vi "get FPS.vi"(8 "error in (no error)":errorcluster, 11 "Thorcam in":refnum<class "Thorcam.lvclass">) -> (0 "error out":errorcluster, 3 "Thorcam out":refnum<class "Thorcam.lvclass">)   [LabVIEW 2012, in "Thorcam.lvclass"]
uses:
  Thorcam.lvclass
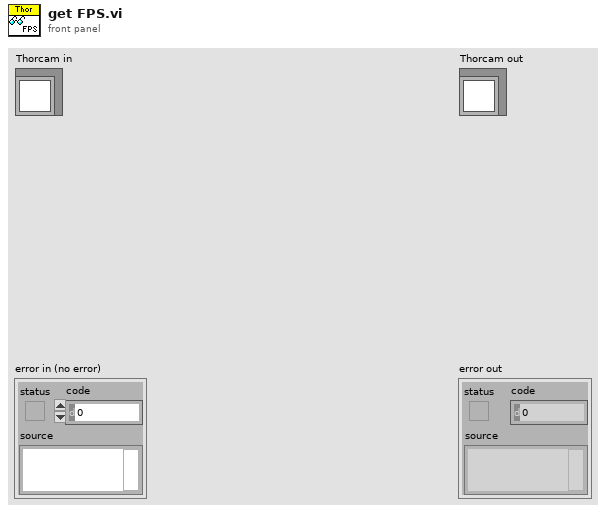
[diagram p1: front panel]
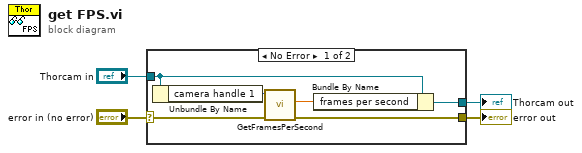
[diagram p0: block diagram]
diagram:
  n1 = case shown="No Error" "error in (no error)" {
    selector: "error in (no error)" -> [w9 w12]
    tunnel: [w8 w12] -> w3
    tunnel: [w6 w11] -> w1
    tunnel: "Thorcam in" -> [w7 w11]
    frame No Error {
      n2 = Unbundle By Name(w7) -> ("camera handle 1"=w10:u32)
      n3 = call <instrlib>:"GetFramesPerSecond.vi"("error in"=w9, "Camera Handle In"=w10) -> ("error out"=w8:errorcluster, "FPS"=w5:dbl)  [unwired: 7 in, 1 out]
      n4 = Bundle By Name(cluster=w7, "frames per second"=w5) -> (w6:refnum<class "Thorcam.lvclass">)
    }
    frame Error {
    }
  }
  "error out" <- w3
  "Thorcam out" <- w1
